vi "Write Value.vi"(8 "error in (no error)":errorcluster, 10 "Data":bool[](array[boolean]), 11 "Boolean in":refnum<class "Const_Bool_1D.lvclass">) -> (0 "error out":errorcluster, 3 "Boolean out":refnum<class "Const_Bool_1D.lvclass">)   [LabVIEW 2021, in "Const_Bool_1D.lvclass"]
uses:
  Const_Bool_1D.lvclass
  Const_Bool_1D.lvclass/Const_Bool_1D.ctl
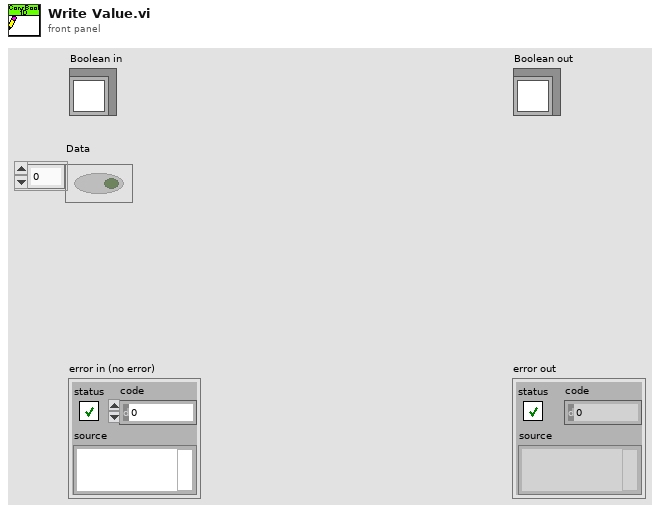
[diagram p1: front panel]
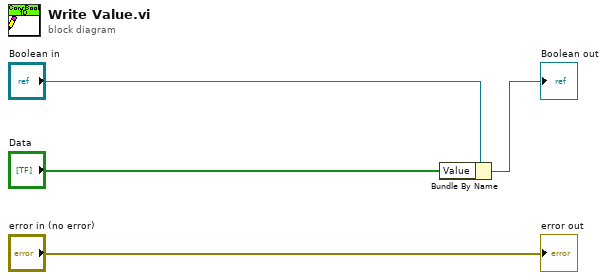
[diagram p0: block diagram]
diagram:
  n1 = Bundle By Name(cluster="Boolean in", "Value"="Data") -> (→"Boolean out":refnum<class "Const_Bool_1D.lvclass">)
  "error out" <- "error in (no error)"
